vi "Durability_will_2012_07_17_main.vi"() -> ()   [LabVIEW 2011]
uses:
  Program Files/National Instruments/LabVIEW 2011/resource/objmgr/daqmx.rc
panel:
  out "error out":errorcluster
  in  "Speed 2/3":i8(slide)=100 min=0 max=100 step=10 scale=0.0..100.0
  in  "Speed 1":i8(slide)=50 min=0 max=100 step=10 scale=0.0..100.0
  in  "Motor 3":bool
  in  "Motor 2":bool
  in  "Motor 1":bool=TRUE
  in  "Quit 4":bool
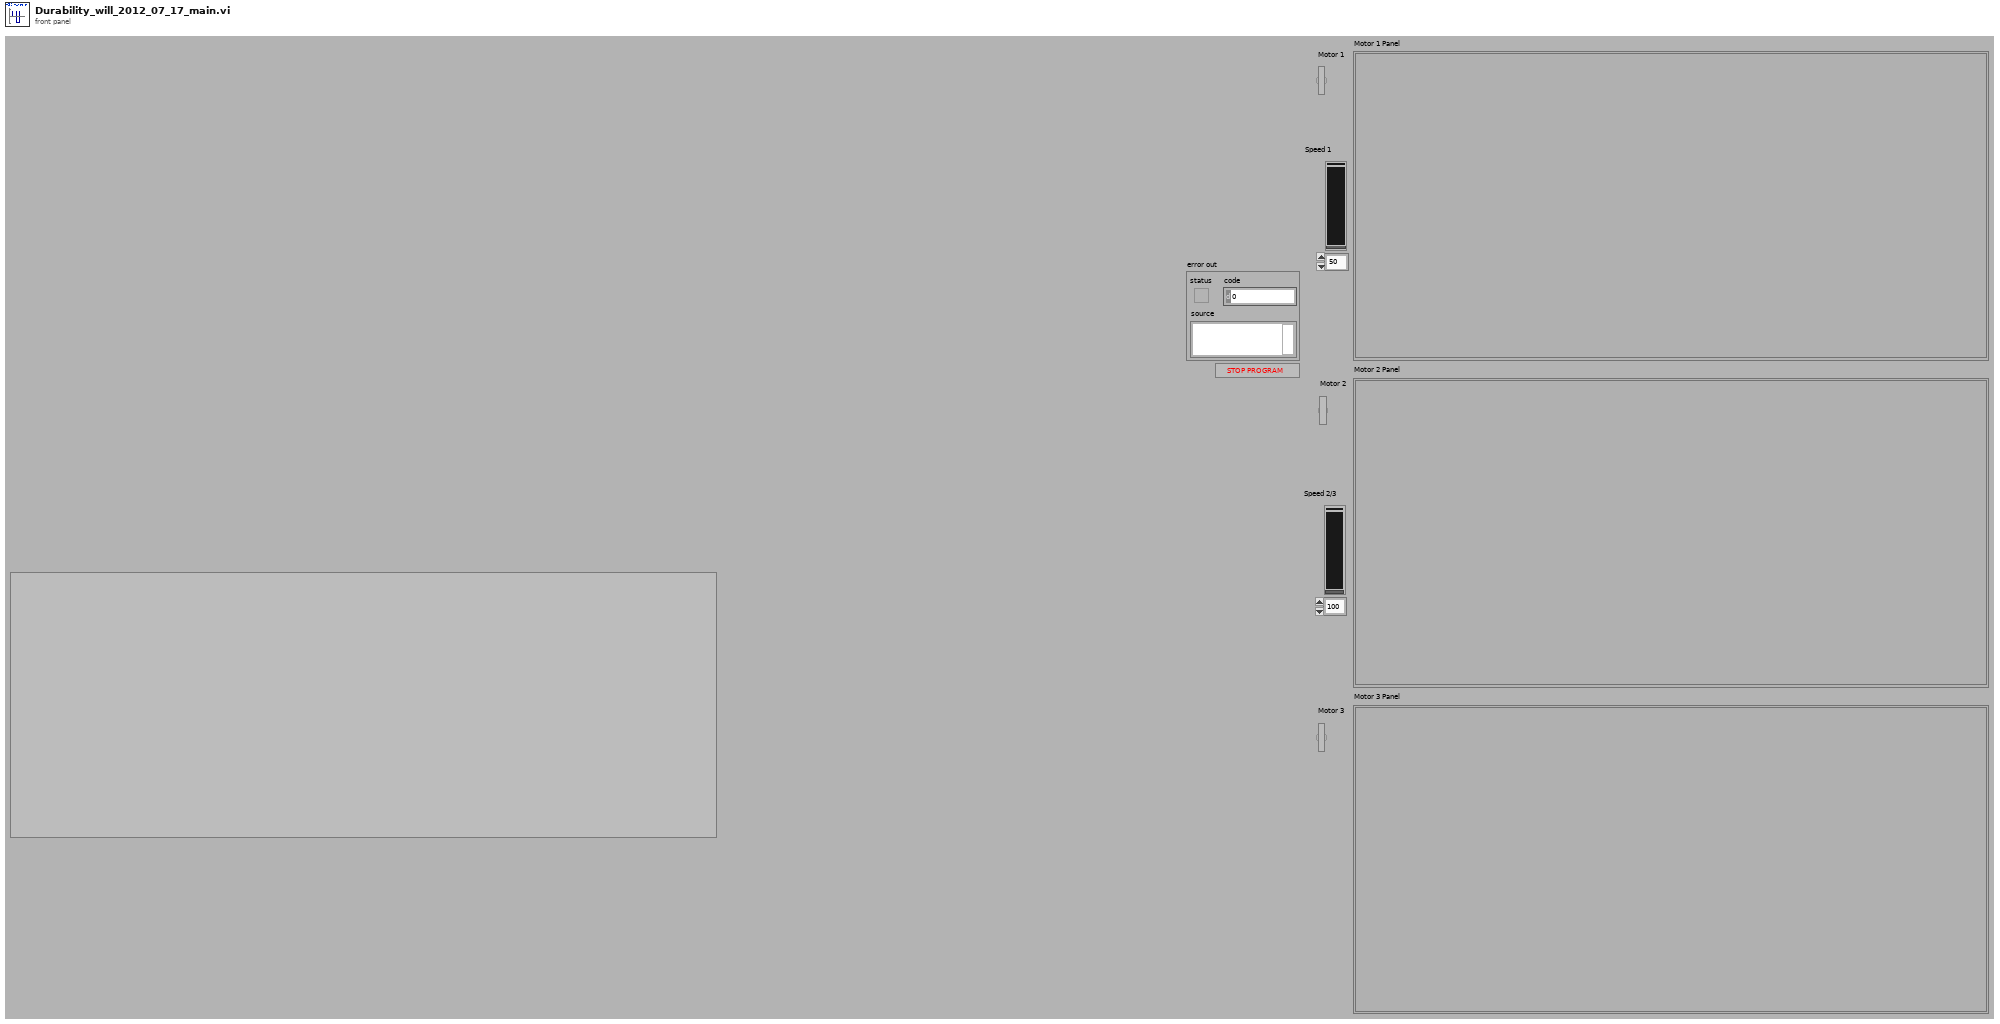
[diagram p1: front panel]
types:
  T1 = enum8{"Enabled", "Disabled", "Disabled and Grayed Out"}
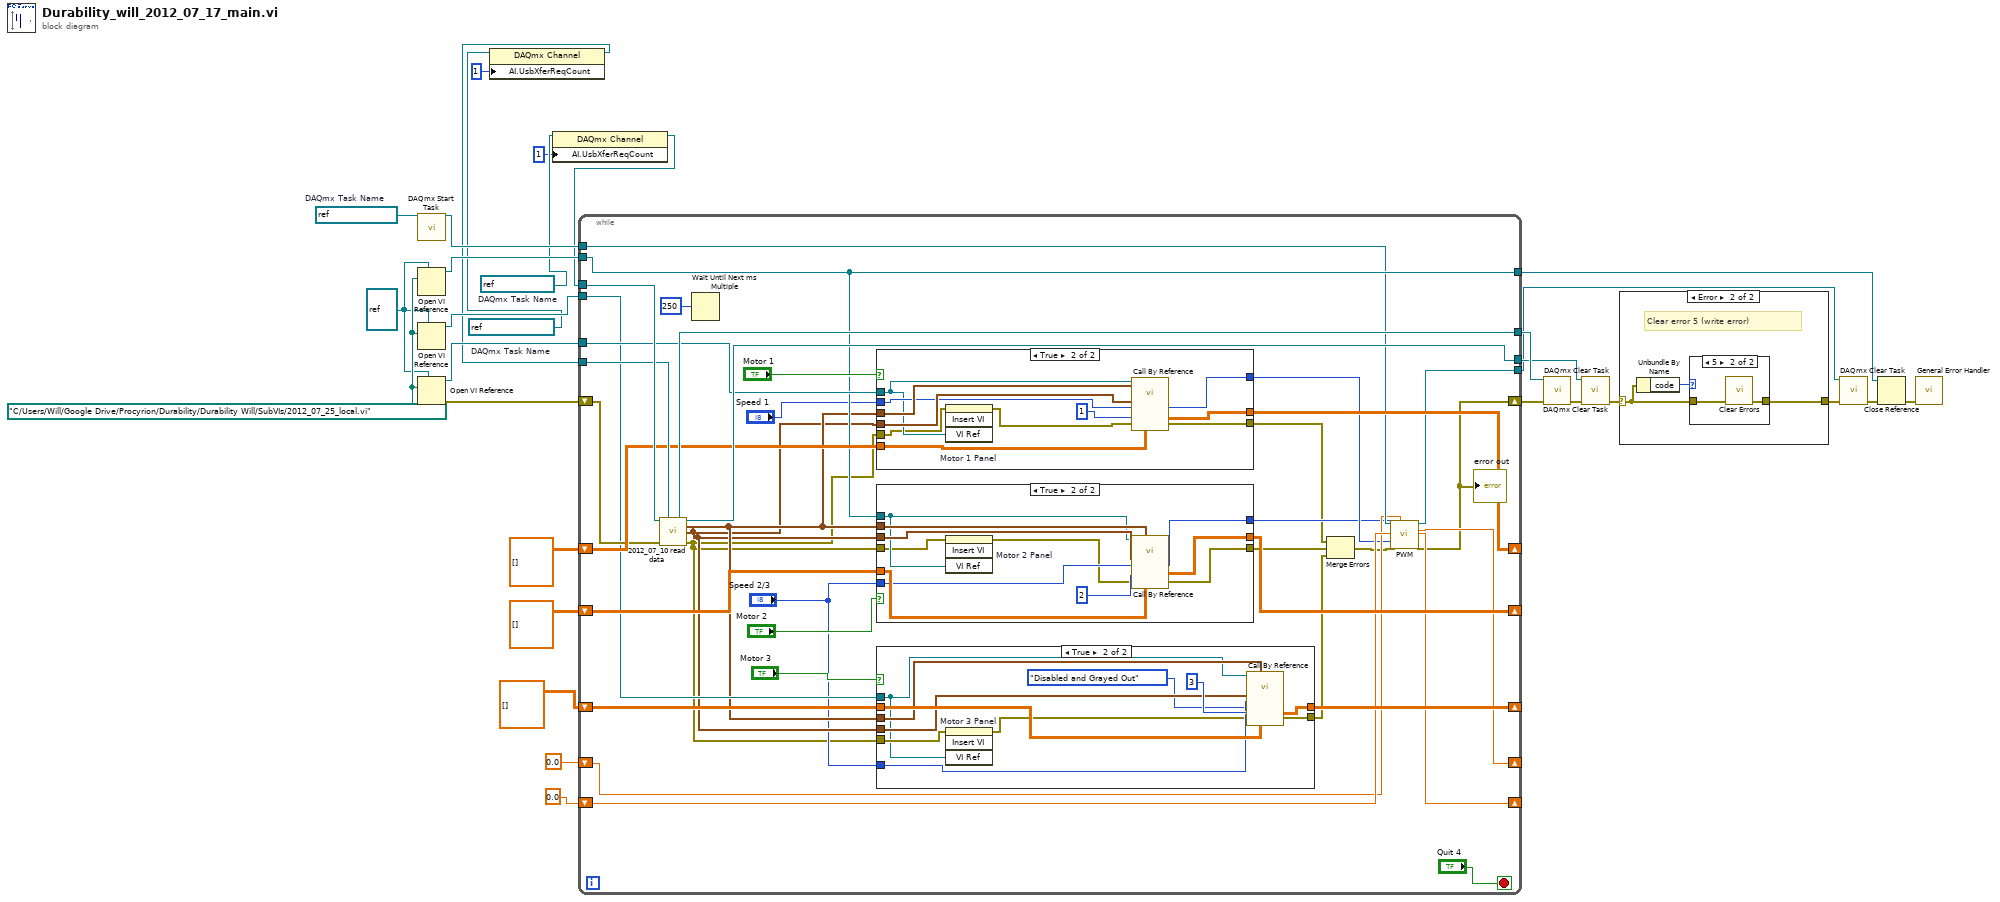
[diagram p0: block diagram]
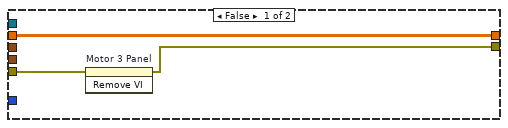
[diagram p4: hidden frame]
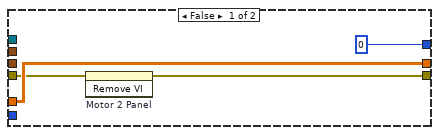
[diagram p5: hidden frame]
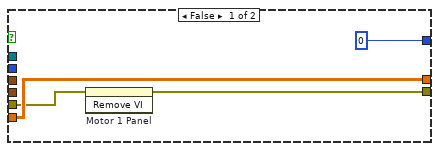
[diagram p6: hidden frame]
diagram:
  w13 = path "C:/Users/Will/Google Drive/Procyrion/Durability/Durability Will/SubVIs/2012_07_25_local.vi" ("'each motor' path")
  w12 = refnum<vi> refnum ("type specifier VI Refnum (for type only)")
  w16 = refnum<k21> "PWM Signal"  # DAQmx Task Name
  w6 = refnum<k21> "MC Power"  # DAQmx Task Name
  w2 = refnum<k21> "Motor Power"  # DAQmx Task Name
  n1 = call <vilib>:"DAQmx Start Task.vi"("task/channels in"=w16) -> ("task out"=w14:refnum<k21>)  [unwired: 13 in, 1 out]
  n2 = Open VI Reference(type specifier VI Refnum (for type only)=w12, vi path=w13) -> (vi reference=w8:refnum<vi>)  [unwired: 4 in, 1 out]
  n3 = Open VI Reference(type specifier VI Refnum (for type only)=w12, vi path=w13) -> (vi reference=w7:refnum<vi>)  [unwired: 4 in, 1 out]
  n4 = Open VI Reference(type specifier VI Refnum (for type only)=w12, vi path=w13) -> (vi reference=w9:refnum<vi>, error out=w15:errorcluster)  [unwired: 4 in]
  n5 = property class="DAQmx Channel"(reference=w2, "AI.UsbXferReqCount"=u32 1) -> (reference out=w1:refnum<k21>)  [unwired: 1 in, 1 out]
  n6 = property class="DAQmx Channel"(reference=w6, "AI.UsbXferReqCount"=u32 1) -> (reference out=w5:refnum<k21>)  [unwired: 1 in, 1 out]
  n7 = while {
    tunnel: w5 -> [w64]
    tunnel: w1 -> [w63]
    shift-right: [w59] -> _
    shift-left: dbl[][][] [] -> [w60]
    shift-right: [w32] -> w29
    shift-left: w15 -> [w52]
    shift-right: [w39] -> _
    shift-left: 0.0 -> [w40]
    tunnel: [w62] -> w23
    tunnel: [w61] -> w22
    shift-right: [w56] -> _
    shift-left: dbl[][][] [] -> [w57]
    shift-right: [w38] -> _
    shift-left: 0.0 -> [w41]
    tunnel: w9 -> [w55]
    tunnel: [w53] -> w19
    tunnel: w8 -> [w53]
    tunnel: w14 -> [w51]
    shift-right: [w50] -> _
    shift-left: dbl[][][] [] -> [w49]
    tunnel: w7 -> [w48]
    tunnel: [w44] -> w11
    stop <- "Quit 4" stop-if-true
    n8 = call "2012_07_10 read data.vi"("MC Power"=w64, "Motor Power"=w63, "Error In"=w52) -> ("Motor Power Out"=w62:refnum<k21>, "MC Power Out"=w61:refnum<k21>, "Motor Power Data"=w46:waveform(dbl)[], "MC Power Data"=w45:waveform(dbl)[], "error out"=w35:errorcluster)  [unwired: 8 in]
    n9 = Wait Until Next ms Multiple(millisecond multiple=u32 250) -> ()  [unwired: 1 out]
    n10 = case shown="True" "Motor 1" {
      tunnel: [w97 w105] -> w30
      tunnel: w35 -> [w96 w101]
      tunnel: w60 -> [w99 w109]
      tunnel: [w99 w110] -> w59
      tunnel: w45 -> [_ w107]
      tunnel: w46 -> [_ w106]
      tunnel: w55 -> [_ w102]
      tunnel: "Speed 1" -> [_ w104]
      tunnel: [i8 0 ("Power \nSetting") w103] -> w37
      frame False {
        n11 = invoke on="Motor 1 Panel" class="SubPnl" method="Remove VI"(error in=w96) -> (error out=w97:errorcluster)  [unwired: 2 in, 2 out]
      }
      frame True {
        n12 = invoke on="Motor 1 Panel" class="SubPnl" method="Insert VI"(error in=w101, "VI Ref"=w102) -> (error out=w100:errorcluster)  [unwired: 2 in, 3 out]
        n13 = call-by-ref "?"(reference=w102, "MC Power Data In"=w107, "Motor Power Data In"=w106, "Power \nSetting"=w104, "Motor"=i16 1, "Error In"=w100, "Fine Data In"=w109) -> ("Power \nSetting"=w103:i8, "Fine Data Out"=w110:dbl[][][], "Errors"=w105:errorcluster)  [unwired: 8 in, 2 out]
      }
    }
    n14 = case shown="True" "Motor 2" {
      tunnel: [w82 w95] -> w31
      tunnel: w57 -> [w84 w93]
      tunnel: [w84 w94] -> w56
      tunnel: w53 -> [_ w87]
      tunnel: w45 -> [_ w91]
      tunnel: w46 -> [_ w90]
      tunnel: w35 -> [w81 w86]
      tunnel: "Speed 2/3" -> [_ w89]
      tunnel: [i8 0 ("Power \nSetting") w88] -> w36
      frame False {
        n15 = invoke on="Motor 2 Panel" class="SubPnl" method="Remove VI"(error in=w81) -> (error out=w82:errorcluster)  [unwired: 2 in, 2 out]
      }
      frame True {
        n16 = invoke on="Motor 2 Panel" class="SubPnl" method="Insert VI"(error in=w86, "VI Ref"=w87) -> (error out=w85:errorcluster)  [unwired: 2 in, 3 out]
        n17 = call-by-ref "?"(reference=w87, "MC Power Data In"=w91, "Motor Power Data In"=w90, "Power \nSetting"=w89, "Motor"=i16 2, "Error In"=w85, "Fine Data In"=w93) -> ("Power \nSetting"=w88:i8, "Fine Data Out"=w94:dbl[][][], "Errors"=w95:errorcluster)  [unwired: 8 in, 2 out]
      }
    }
    n18 = case shown="True" "Motor 3" {
      tunnel: [w67 w80] -> w34
      tunnel: w49 -> [w69 w78]
      tunnel: [w69 w79] -> w50
      tunnel: w48 -> [_ w70]
      tunnel: w45 -> [_ w76]
      tunnel: w46 -> [_ w75]
      tunnel: w35 -> [w68 w72]
      tunnel: "Speed 2/3" -> [_ w74]
      frame False {
        n19 = invoke on="Motor 3 Panel" class="SubPnl" method="Remove VI"(error in=w68) -> (error out=w67:errorcluster)  [unwired: 2 in, 2 out]
      }
      frame True {
        n20 = invoke on="Motor 3 Panel" class="SubPnl" method="Insert VI"(error in=w72, "VI Ref"=w70) -> (error out=w71:errorcluster)  [unwired: 2 in, 3 out]
        n21 = call-by-ref "?"(reference=w70, "MC Power Data In"=w76, "Motor Power Data In"=w75, "Power \nSetting"=w74, "On/Off Control"=T1."Disabled and Grayed Out", "Motor"=i16 3, "Error In"=w71, "Fine Data In"=w78) -> ("Fine Data Out"=w79:dbl[][][], "Errors"=w80:errorcluster)  [unwired: 7 in, 3 out]
      }
    }
    n22 = Merge Errors(w30, w31, w34) -> (w33:errorcluster)
    n23 = call "PWM.vi"("Refnum in"=w51, "High Time In 2"=w41, "Speed 1"=w37, "Speed 2/3"=w36, "error in (no error)"=w33, "High Time In 1"=w40) -> ("Refnum out"=w44:refnum<k21>, "High Time Out 1"=w39:dbl, "High Time Out 2"=w38:dbl, "error out"=w32:errorcluster)  [unwired: 18 in]
    "error out" <- w32
  }
  n24 = call <vilib>:"DAQmx Clear Task.vi"("task in"=w23, "error in"=w29) -> ("error out"=w25:errorcluster)  [unwired: 13 in]
  n25 = call <vilib>:"DAQmx Clear Task.vi"("task in"=w22, "error in"=w25) -> ("error out"=w27:errorcluster)  [unwired: 13 in]
  n26 = case shown="Error" w27 {
    selector: w27 -> [w111 w113]
    tunnel: [w111 w112] -> w26
    frame No Error {
    }
    frame Error {
      # "Clear error 5 (write error)"
      n27 = Unbundle By Name(w113) -> ("code"=w114:i32)
      n28 = case shown="5" w114 {
        tunnel: w113 -> [w115 w117]
        tunnel: [w115 w116] -> w112
        frame Default {
        }
        frame 5 {
          n29 = call <vilib>:"Clear Errors.vi"("error in (no error)"=w117) -> ("error out"=w116:errorcluster)  [unwired: 6 in]
        }
      }
    }
  }
  n30 = call <vilib>:"DAQmx Clear Task.vi"("task in"=w11, "error in"=w26) -> ("error out"=w18:errorcluster)  [unwired: 13 in]
  n31 = Close Reference(reference=w19, error in (no error)=w18) -> (error out=w17:errorcluster)
  n32 = call <vilib>:"General Error Handler.vi"("error in (no error)"=w17) -> ()  [unwired: 10 in, 5 out]
